vi "control.vi"() -> ()   [LabVIEW 2020]
uses:
  <vilib>/Analysis/baseanly.llb/Real A x B.vi
  <vilib>/Analysis/Matrix/Numeric/Conversions/Matrix To Array - RM.vi
  <vilib>/Analysis/NI_AALBase.lvlib
  <vilib>/Analysis/Matrix/NI_Matrix.lvlib
panel:
  in  "num of col for B (p)":i32=1
  in  "num of col for A (n)":i32=7
  in  "num of rows (m)":i32=3
  out "sum of error":dbl
  out "C - FPGA code":sgl[][](array[numeric])
  out "1D array of C":sgl[](array[numeric])
  out "C - Real":dbl[][](array[numeric])
  out "B":dbl[][](array[numeric])
  out "A":dbl[][](array[numeric])
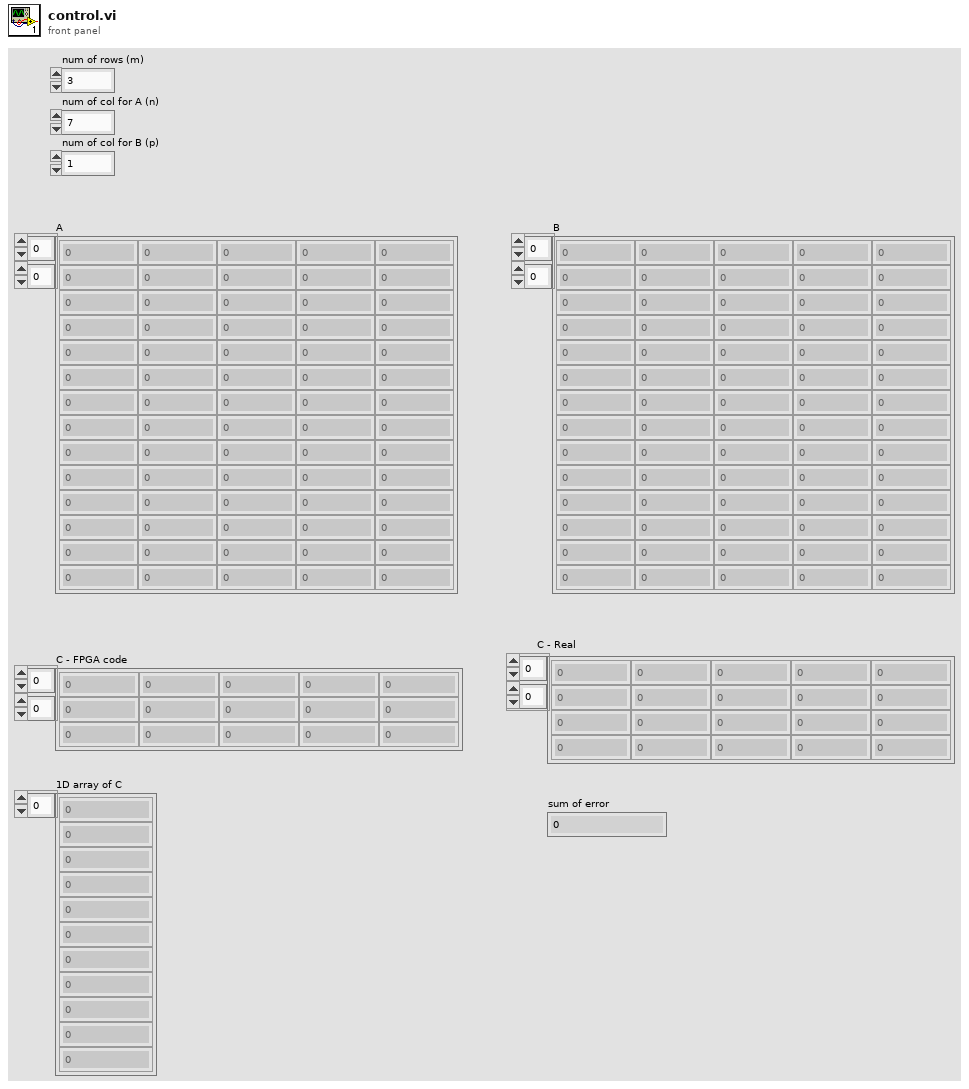
[diagram p1: front panel]
types:
  T1 = typedef "NI_Matrix.lvlib/RealMatrix.ctl" = dbl[][]
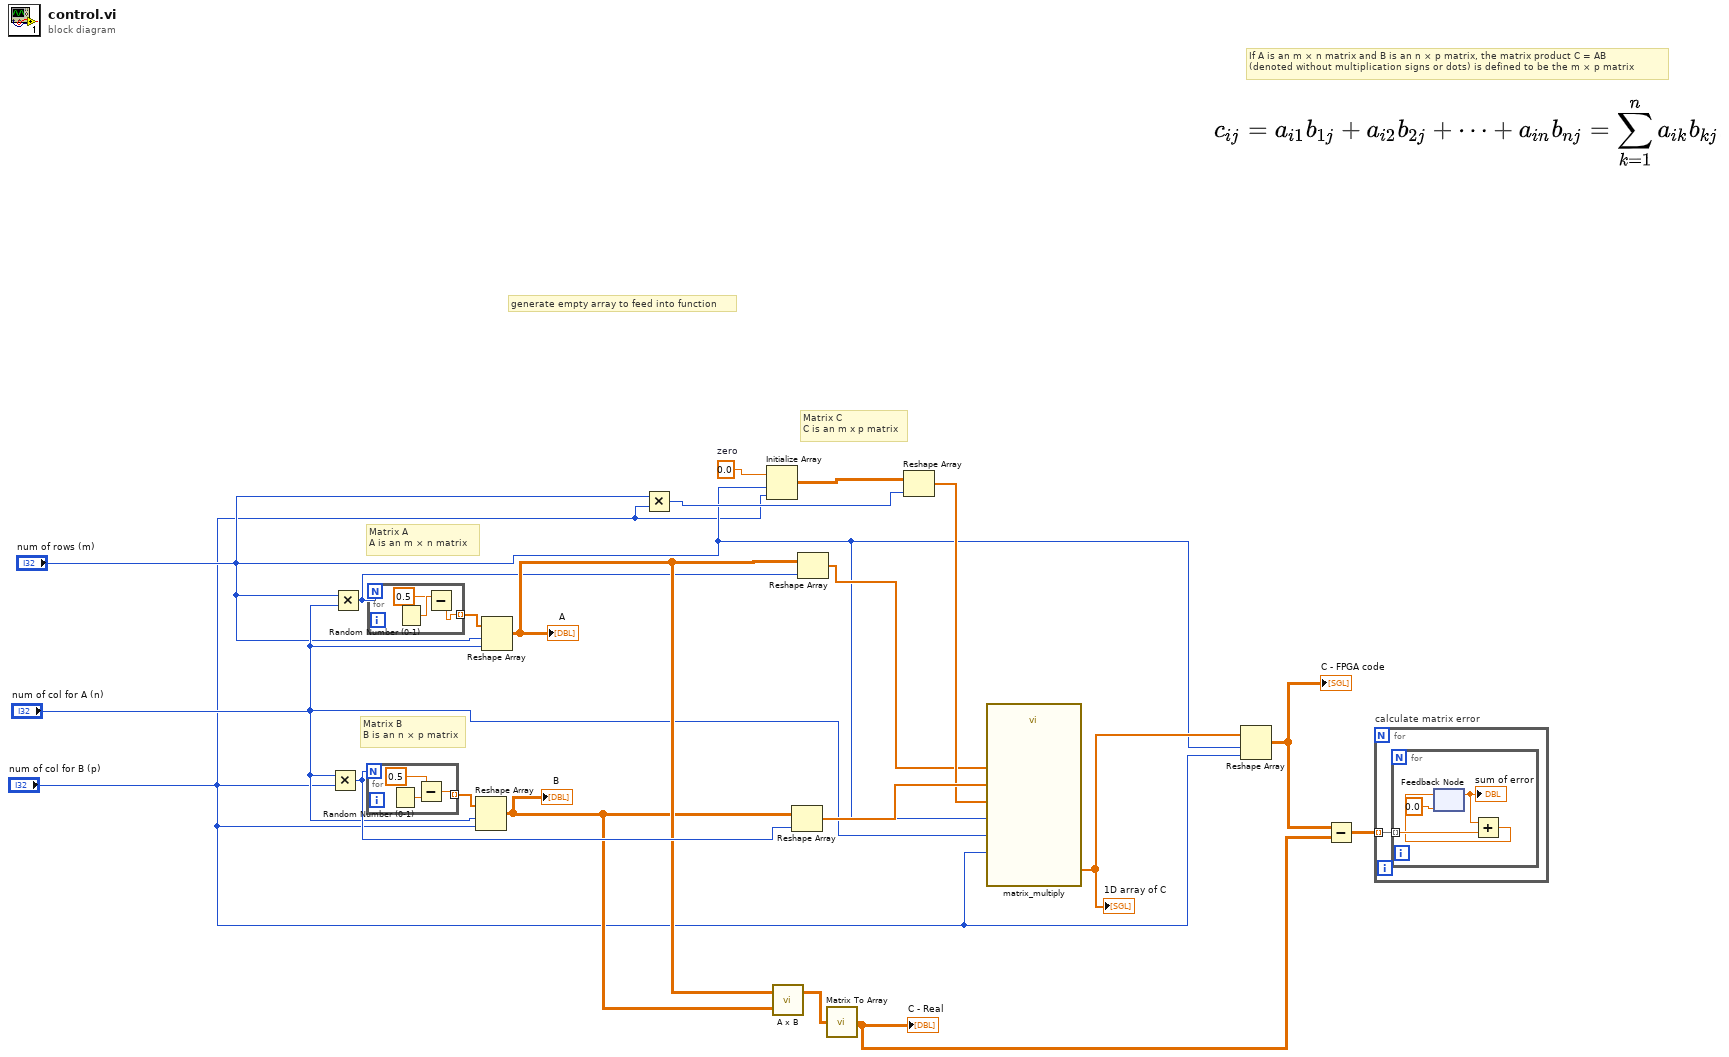
[diagram p0: block diagram]
diagram:
  w17 = sgl 0.0  # zero
  # "Matrix C\nC is an m x p matrix"
  # "If A is an m × n matrix and B is an n × p matrix, the matrix product C = AB \n(denoted without multiplication signs or dots) is defined to be the m × p matrix"
  # "generate empty array to feed into function"
  # "Matrix B\nB is an n × p matrix"
  # "Matrix A\nA is an m × n matrix"
  n1 = Multiply(x="num of col for A (n)", y="num of col for B (p)") -> (x*y=w18:i32)
  n2 = Multiply(x="num of rows (m)", y="num of col for A (n)") -> (x*y=w12:i32)
  n3 = for {
    N: w18 -> [_]
    tunnel: [w22] -> w19 mode=indexing
    n4 = Random Number (0-1)() -> (number: 0 to 1=w23:dbl)
    n5 = Subtract(x=w23, y=0.5) -> (x-y=w22:dbl)
  }
  n6 = for {
    N: w12 -> [_]
    tunnel: [w25] -> w20 mode=indexing
    n7 = Random Number (0-1)() -> (number: 0 to 1=w26:dbl)
    n8 = Subtract(x=w26, y=0.5) -> (x-y=w25:dbl)
  }
  n9 = Reshape Array(w19, "num of col for A (n)", "num of col for B (p)") -> (w15:dbl[][])
  "B" <- w15
  n10 = Reshape Array(w20, "num of rows (m)", "num of col for A (n)") -> (w16:dbl[][])
  "A" <- w16
  n11 = Multiply(x="num of rows (m)", y="num of col for B (p)") -> (x*y=w9:i32)
  n12 = Initialize Array(w17, "num of rows (m)", "num of col for B (p)") -> (w13:sgl[][])
  n13 = call-poly <vilib>:"A x B.vi"("B"=w15, "A"=w16) -> ("A x B"=w14:T1)  [unwired: 1 out]
  n14 = Reshape Array(w15, w18) -> (w11:dbl[])
  n15 = Reshape Array(w16, w12) -> (w7:dbl[])
  n16 = call-poly <vilib>:"Matrix To Array.vi"("Real Matrix"=w14) -> ("Real 2D Array"=w5:dbl[][])
  "C - Real" <- w5
  n17 = Reshape Array(w13, w9) -> (w10:sgl[])
  n18 = call "matrix_multiply.vi"("p"="num of col for B (p)", "C"=w10, "n"="num of col for A (n)", "m"="num of rows (m)", "B"=w11, "A"=w7) -> ("C"=w8:sgl[])
  "1D array of C" <- w8
  n19 = Reshape Array(w8, "num of rows (m)", "num of col for B (p)") -> (w6:sgl[][])
  "C - FPGA code" <- w6
  n20 = Subtract(x=w6, y=w5) -> (x-y=w4:dbl[][])
  n21 = for "calculate matrix error" {
    tunnel: w4 -> [w27] mode=indexing
    n22 = for {
      tunnel: w27 -> [w31] mode=indexing
      n23 = feedback #1(0.0) -> (w29:dbl)
      "sum of error" <- w29
      n24 = Add(x=w29, y=w31) -> (x+y=w30:dbl)
      n25 = feedback-in #1(w30) -> ()
    }
  }
